vi "Ring Set Value and Item Name I64.vi"(8 "error in":errorcluster, 9 "Start Value":i64, 10 "Item Names":string[](array[string]), 11 "Selection Ring Ref in":refnum<vi>) -> (0 "error out":errorcluster, 3 "Selection Ring Ref Out":refnum<vi>)   [LabVIEW 2024]
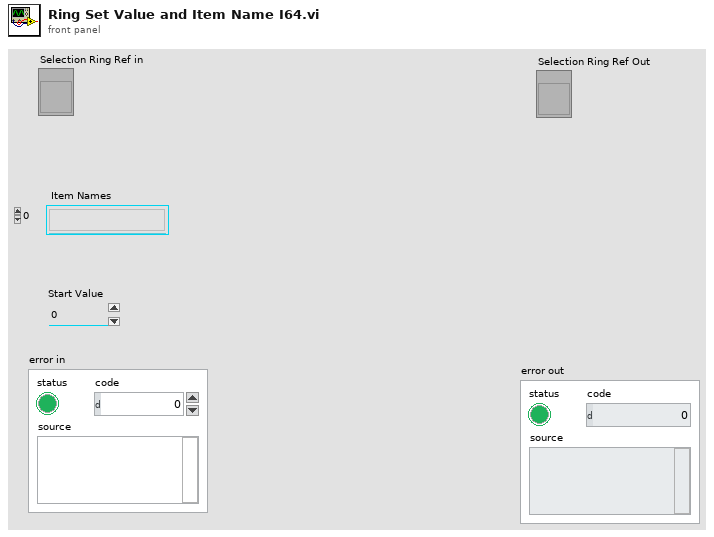
[diagram p1: front panel]
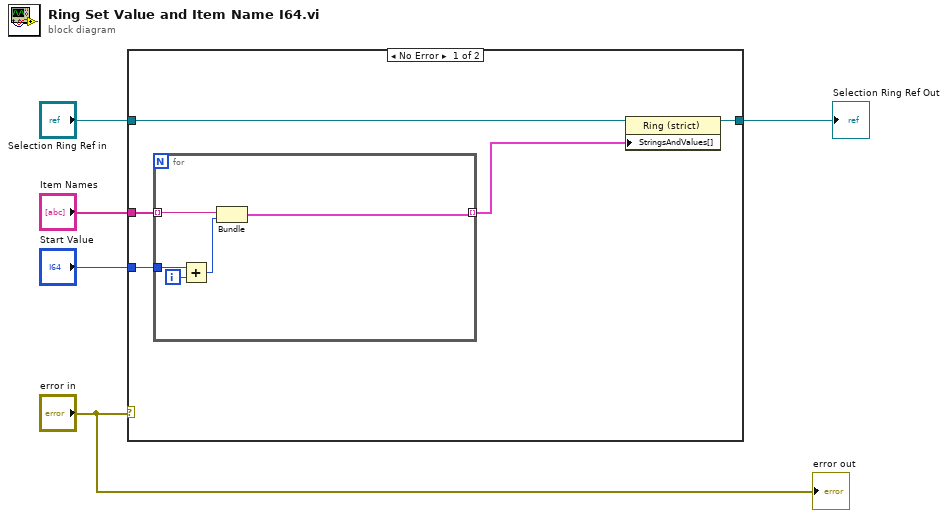
[diagram p0: block diagram]
diagram:
  n1 = case shown="No Error" "error in" {
    tunnel: "Item Names" -> [w10 _]
    tunnel: "Start Value" -> [w9 _]
    tunnel: "Selection Ring Ref in" -> [w8 w16]
    tunnel: [w7 w16] -> w2
    frame No Error {
      n2 = for {
        tunnel: w10 -> [w15] mode=indexing
        tunnel: w9 -> [w14]
        tunnel: [w11] -> w6 mode=indexing
        i -> [w13]
        n3 = Add(x=w14, y=w13) -> (x+y=w12:i64)
        n4 = Bundle("String"=w15, w12) -> (w11:cluster{"String":string, i64})  [unwired: 1 in]
      }
      n5 = property class="Ring (strict)"(reference=w8, "StringsAndValues[]"=w6) -> (reference out=w7:refnum<vi>)  [unwired: 1 in, 1 out]
    }
    frame Error {
    }
  }
  "Selection Ring Ref Out" <- w2
  "error out" <- "error in"
